vi "Show Caller Items Dialog.vi"(6 "Event":refnum<vi>, 8 "Find Broadcast?":bool=TRUE, 9 "Theme":bool, 11 "Request VI Callers":refnum<vi>[](array[refnum])) -> ()   [LabVIEW 2019, in "Panther Dashboard.lvlib"]
uses:
  Panther Dashboard.lvlib
  <vilib>/Utility/traverseref.llb/TRef TravTarget.ctl
  <vilib>/Utility/traverseref.llb/VI Scripting - Traverse.lvlib
panel:
  in  "Results Listbox":i32(listbox)
  # "» Double click an element to navigate into code\n» Right-click event to find the file on disk"
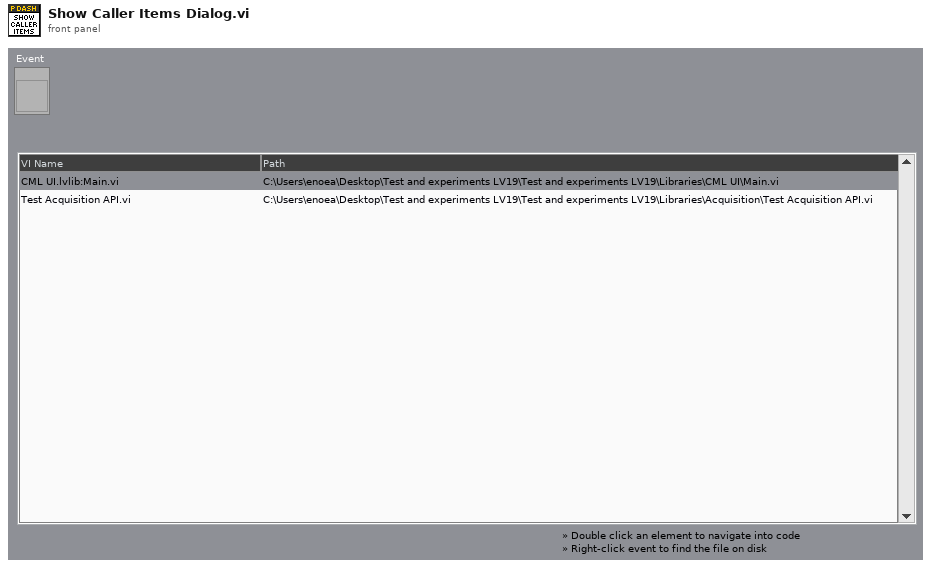
[diagram p1: front panel]
types:
  T1 = typedef "TRef TravTarget.ctl" = enum16{"FP", "BD", "Other"}
  T2 = typedef "LVRowAndColumnTypeDef.ctl" = cluster{"Row":i32, "Column":i32}
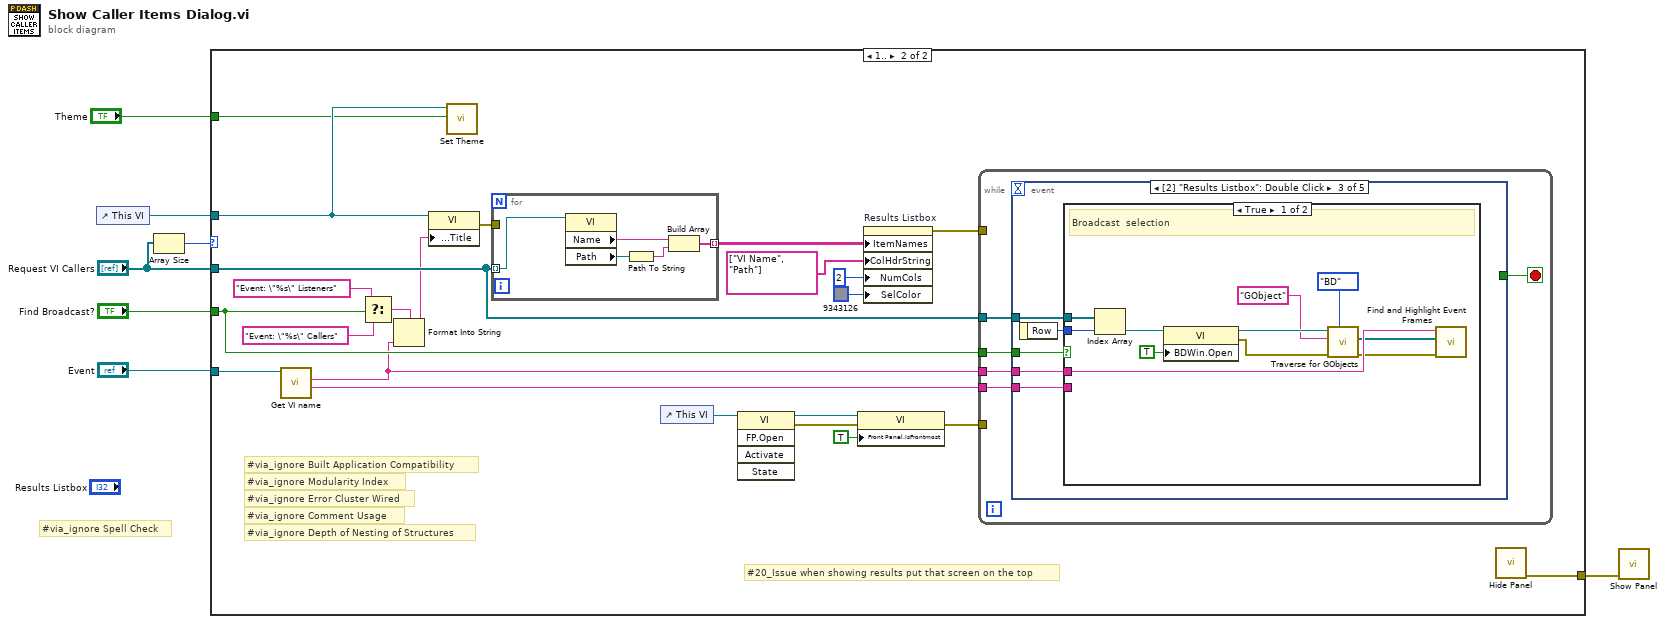
[diagram p0: block diagram]
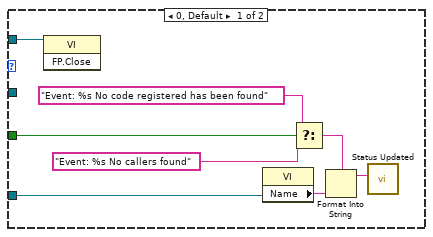
[diagram p2: hidden frame]
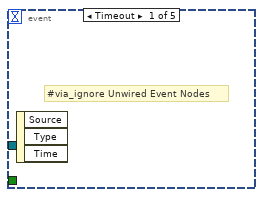
[diagram p3: hidden frame]
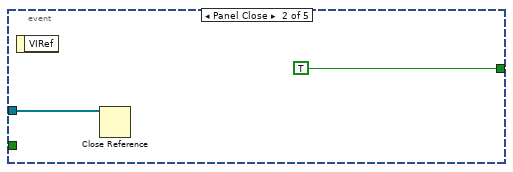
[diagram p4: hidden frame]
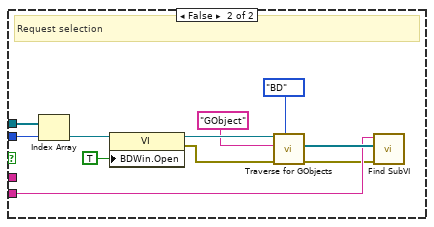
[diagram p5: hidden frame]
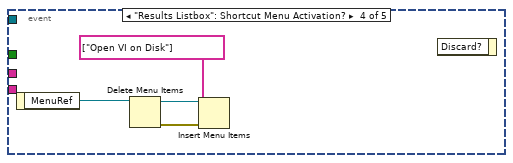
[diagram p6: hidden frame]
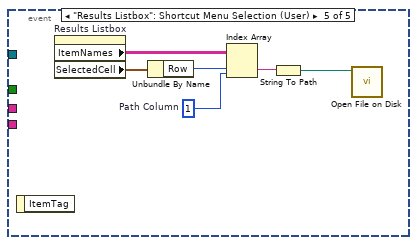
[diagram p7: hidden frame]
diagram:
  # "#via_ignore Spell Check"
  n1 = control-ref of="This VI"() -> (w2:refnum<vi>)
  n2 = Array Size(array="Request VI Callers") -> (size(s)=w6:i32)
  n3 = case shown="1.." w6 {
    tunnel: "Request VI Callers" -> [_ w30]
    tunnel: "Event" -> [w13 w27]
    tunnel: "Find Broadcast?" -> [w12 w29]
    tunnel: "Theme" -> [_ w22]
    tunnel: w2 -> [w8 w24]
    tunnel: [_ w20] -> w1
    frame 0, Default {
      n4 = invoke class="VI" method="FP.Close"(reference=w8) -> ()  [unwired: 2 in, 3 out]
      n5 = property class="VI"(reference=w13) -> ("Name"=w14:string)  [unwired: 1 in, 2 out]
      n6 = Select(t="Event: %s No code registered has been found" ("Origin"), s=w12, f="Event: %s No callers found" ("Origin")) -> (s? t:f=w10:string)
      n7 = Format Into String(format string=w10, w14) -> (resulting string=w15:string)  [unwired: 2 in, 1 out]
      n8 = call "Status Updated.vi"("Status"=w15) -> ()  [unwired: 10 in, 1 out]
    }
    frame 1.. {
      # "#20_Issue when showing results put that screen on the top"
      # "#via_ignore Built Application Compatibility"
      # "#via_ignore Modularity Index"
      # "#via_ignore Depth of Nesting of Structures"
      # "#via_ignore Error Cluster Wired"
      # "#via_ignore Comment Usage"
      n9 = call "Get VI name.vi"("VI in"=w27) -> ("Full Vi Name"=w25:string, "Plain Name"=w26:string)  [unwired: 8 in, 1 out]
      n10 = Select(t="Event: \"%s\" Listeners" ("Origin"), s=w29, f="Event: \"%s\" Callers" ("Origin")) -> (s? t:f=w32:string)
      n11 = Format Into String(format string=w32, w26) -> (resulting string=w21:string)  [unwired: 2 in, 1 out]
      n12 = property class="VI"(reference=w24, "Front Panel.Title"=w21) -> (error out=w37:errorcluster)  [unwired: 1 in, 1 out]
      n13 = call "Set Theme.vi"("Dark?"=w22, "VI in"=w24) -> ()  [unwired: 10 in]
      n14 = for {
        tunnel: w30 -> [w43] mode=indexing
        tunnel: [w39] -> w36 mode=indexing
        tunnel: w37 -> [_]
        n15 = property class="VI"(reference=w43) -> ("Name"=w42:string, "Path"=w41:path)  [unwired: 1 in, 2 out]
        n16 = Path To String(path=w41) -> (string=w40:string)
        n17 = Build Array(w42, w40) -> (w39:string[])
      }
      n18 = control-ref of="This VI"() -> (w19:refnum<vi>)
      n19 = invoke class="VI" method="FP.Open"(reference=w19) -> (reference out=w17:refnum<vi>, error out=w28:errorcluster)  [unwired: 4 in, 3 out]
      n20 = property class="VI"(reference=w17, error in=w28, "Front Panel.IsFrontmost"=TRUE ("Front Panel Window:Is Frontmost")) -> (error out=w18:errorcluster)  [unwired: 1 out]
      n21 = property on="Results Listbox" class="MCListbox (strict)"("ItemNames"=w36, "ColHdrString"=string[] ["VI Name", "Path"] ("Column Header Strings[]"), "NumCols"=u32 2 ("Number of Columns"), "SelColor"=u32 9343126) -> (error out=w38:errorcluster)  [unwired: 2 in, 1 out]
      n22 = while {
        tunnel: w30 -> [w48]
        tunnel: w38 -> [_]
        tunnel: w29 -> [w46]
        tunnel: w26 -> [w45]
        tunnel: w18 -> [_]
        tunnel: w25 -> [w44]
        stop <- w47 stop-if-true
        n23 = event shown="[2] \"Results Listbox\": Double Click" {
          selector: _ -> [_ _ _ _ _]
          dyn-events: _ -> [_ _ _ _ _]
          timeout: _ -> [_ _ _ _ _]
          tunnel: w48 -> [_ w50 w55 _ _]
          tunnel: [_ TRUE _ _ _] -> w47
          tunnel: w46 -> [_ _ w53 _ _]
          tunnel: w45 -> [_ _ w52 _ _]
          tunnel: w44 -> [_ _ w51 _ _]
          event Timeout {
            # "#via_ignore Unwired Event Nodes"
            n24 = event-data() -> ()  [unwired: 1 in, 3 out]
          }
          event Panel Close {
            n25 = event-data() -> ()  [unwired: 1 in, 1 out]
            n26 = Close Reference(reference=w50) -> ()  [unwired: 1 in, 1 out]
          }
          event "Results Listbox": Double Click {
            n27 = event-data() -> ("Row"=w54:i32)  [unwired: 1 in]
            n28 = case shown="True" w53 {
              tunnel: w55 -> [w65 w76]
              tunnel: w54 -> [w64 w75]
              tunnel: w52 -> [w59 _]
              tunnel: w51 -> [_ w69]
              frame True {
                # "Broadcast  selection"
                n29 = Index Array(array=w65, index=w64) -> (element=w60:refnum<vi>)
                n30 = property class="VI"(reference=w60, "BDWin.Open"=TRUE ("Block Diagram Window:Open")) -> (reference out=w63:refnum<vi>, error out=w57:errorcluster)  [unwired: 1 in]
                n31 = call <vilib>:"Traverse for GObjects.vi"("Traverse Target"=TRef_TravTarget."BD", "error in (no error)"=w57, "Class Name"="GObject", "VI Refnum"=w63) -> ("error out"=w56:errorcluster, "References"=w58:refnum<vi>[])  [unwired: 4 in, 2 out]
                n32 = call "Find and Highlight Event Frames.vi"("error in"=w56, "References"=w58, "Event Name"=w59) -> ()  [unwired: 8 in, 1 out]
              }
              frame False {
                # "Request selection"
                n33 = Index Array(array=w76, index=w75) -> (element=w71:refnum<vi>)
                n34 = property class="VI"(reference=w71, "BDWin.Open"=TRUE ("Block Diagram Window:Open")) -> (reference out=w74:refnum<vi>, error out=w68:errorcluster)  [unwired: 1 in]
                n35 = call <vilib>:"Traverse for GObjects.vi"("Traverse Target"=TRef_TravTarget."BD", "error in (no error)"=w68, "Class Name"="GObject", "VI Refnum"=w74) -> ("error out"=w67:errorcluster, "References"=w70:refnum<vi>[])  [unwired: 4 in, 2 out]
                n36 = call "Find SubVI.vi"("error in"=w67, "References"=w70, "Full Vi Name"=w69) -> ()  [unwired: 8 in, 1 out]
              }
            }
          }
          event "Results Listbox": Shortcut Menu Activation? {
            n37 = event-data() -> ("MenuRef"=w81:refnum<k9>)  [unwired: 1 in]
            n38 = Delete Menu Items(9:w81) -> (0:w79:errorcluster, 3:w80:refnum<k9>)  [unwired: 3 in]
            n39 = Insert Menu Items(6:w79, 8:string[] ["Open VI on Disk"] ("item names"), 9:w80) -> ()  [unwired: 3 in, 3 out]
            n40 = event-data() -> ()  [unwired: 2 in, 1 out]
          }
          event "Results Listbox": Shortcut Menu Selection (User) {
            w84 = 1  # Path Column
            n41 = event-data() -> ()  [unwired: 1 in, 1 out]
            n42 = property on="Results Listbox" class="MCListbox (strict)"() -> ("ItemNames"=w87:string[][], "SelectedCell"=w86:T2)  [unwired: 2 in, 2 out]
            n43 = Unbundle By Name(w86) -> ("Row"=w85:i32)
            n44 = Index Array(array=w87, index (row)=w85, index (col)=w84) -> (element=w83:string)
            n45 = String To Path(string=w83) -> (path=w82:path)
            n46 = call "Open File on Disk.vi"("file or directory path"=w82) -> ()  [unwired: 10 in, 1 out]
          }
        }
      }
      n47 = call "Hide Panel.vi"() -> ("error out"=w20:errorcluster)  [unwired: 11 in]
    }
  }
  n48 = call "Show Panel.vi"("error in (no error)"=w1) -> ()  [unwired: 10 in, 1 out]
